vi "Execute.vi"(8 "error in (no error)":errorcluster, 11 "Console Wrapper in":refnum<class "Console Wrapper.lvclass">) -> (0 "error out":errorcluster, 2 "Command output":string, 3 "Console Wrapper out":refnum<class "Console Wrapper.lvclass">)   [LabVIEW 2020, in "Console Wrapper.lvclass"]
doc: "This method defines the steps for excuting a command:\n\n1. It builds a command - Default implementation\n2. it runs the command - Default implementation\n3. It process the Standard Output - Abstract Method."
uses:
  Console Wrapper.lvclass
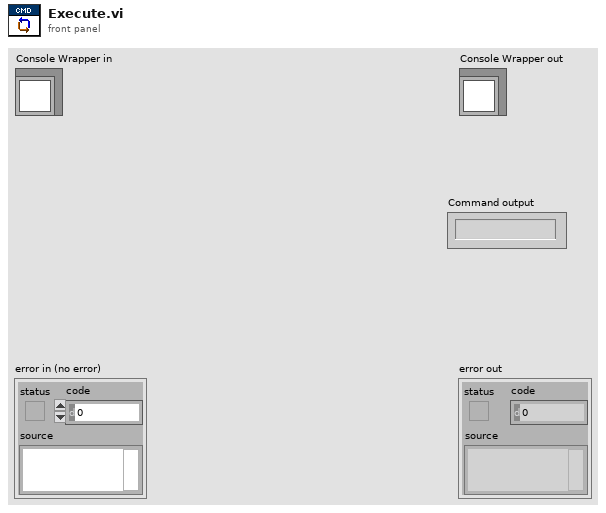
[diagram p1: front panel]
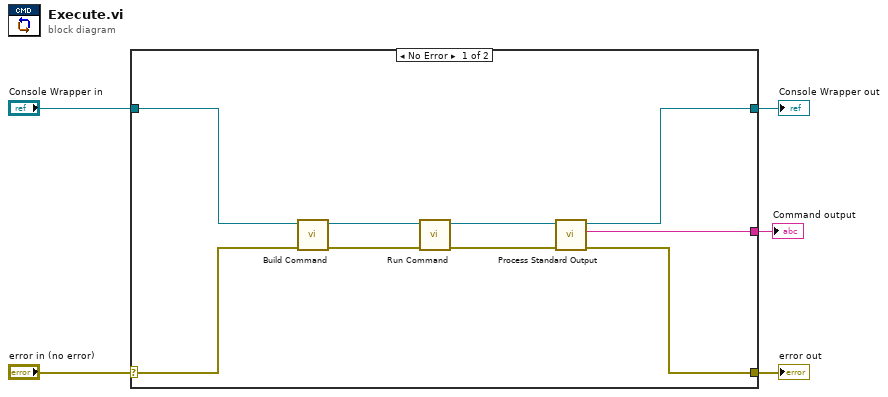
[diagram p0: block diagram]
diagram:
  n1 = case shown="No Error" "error in (no error)" {
    selector: "error in (no error)" -> [w14 w16]
    tunnel: [w9 w16] -> w4
    tunnel: [w7 w15] -> w2
    tunnel: "Console Wrapper in" -> [w12 w15]
    tunnel: [w6 _] -> w1
    frame No Error {
      n2 = call "Build Command.vi"("error in (no error)"=w14, "Console Wrapper in"=w12) -> ("error out"=w13:errorcluster, "Console Wrapper out"=w10:refnum<class "Console Wrapper.lvclass">)  [unwired: 8 in]
      n3 = call "Run Command.vi"("error in (no error)"=w13, "Console Wrapper in"=w10) -> ("error out"=w11:errorcluster, "Console Wrapper out"=w8:refnum<class "Console Wrapper.lvclass">)  [unwired: 8 in]
      n4 = call-dynamic "Process Standard Output.vi"("error in (no error)"=w11, "Console Wrapper in"=w8) -> ("error out"=w9:errorcluster, "Command output"=w6:string, "Console Wrapper out"=w7:refnum<class "Console Wrapper.lvclass">)  [unwired: 7 in]
    }
    frame Error {
    }
  }
  "error out" <- w4
  "Console Wrapper out" <- w2
  "Command output" <- w1
